vi "Power_Scale_Line.vi"(1 "Power Input":dbl, 2 "POV":i16) -> (0 "Power Output":dbl)   [LabVIEW 2015]
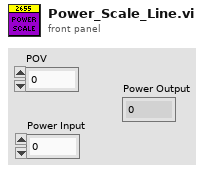
[diagram p1: front panel]
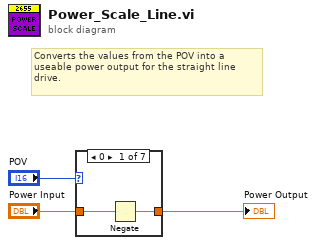
[diagram p0: block diagram]
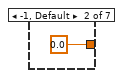
[diagram p2: hidden frame]
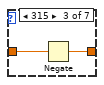
[diagram p3: hidden frame]
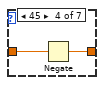
[diagram p4: hidden frame]
diagram:
  # "Converts the values from the POV into a useable power output for the straight line drive."
  n1 = case shown="0" "POV" {
    tunnel: [w5 0.0 w8 w10 w11 w12 w13] -> w2
    tunnel: "Power Input" -> [w4 _ w7 w9 w11 w12 w13]
    frame 0 {
      n2 = Negate(x=w4) -> (-x=w5:dbl)
    }
    frame -1, Default {
    }
    frame 315 {
      n3 = Negate(x=w7) -> (-x=w8:dbl)
    }
    frame 45 {
      n4 = Negate(x=w9) -> (-x=w10:dbl)
    }
    frame 135 {
    }
    frame 180 {
    }
    frame 225 {
    }
  }
  "Power Output" <- w2
